vi "array.vi"() -> ()   [LabVIEW 2018]
panel:
  in  "数组 4":bool[](array[boolean])
  in  "数组 3":dbl[][](array[numeric])
  out "数组函数":i32[](array[numeric])
  in  "停止":bool
  out "数组 2":i32[](array[numeric])
  out "数组":i32[](array[numeric])
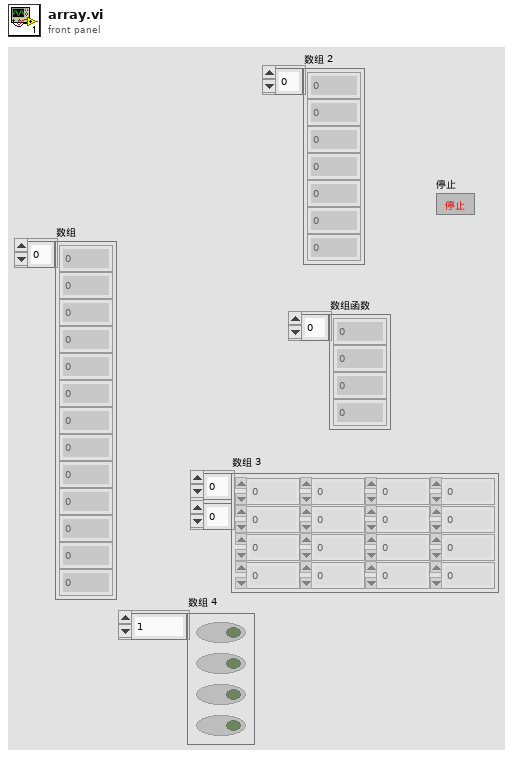
[diagram p1: front panel]
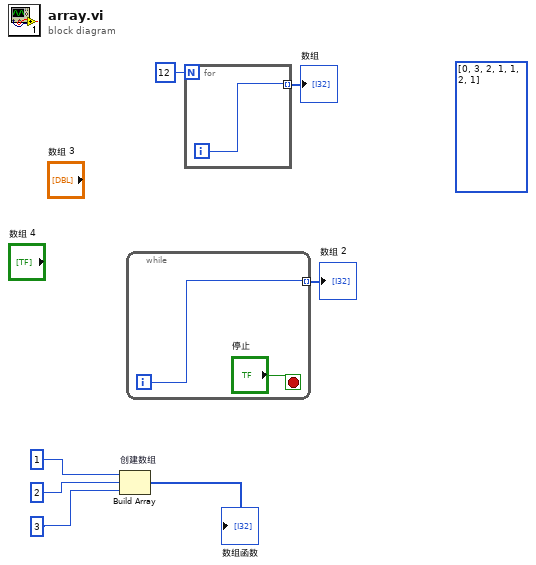
[diagram p0: block diagram]
diagram:
  (unwired) i32[] [0, 3, 2, 1, 1, 2, 1]
  n1 = Build Array "创建数组"(1, 2, 3) -> (→"数组函数":i32[])
  n2 = while {
    tunnel: [w9] -> w5 mode=indexing
    i -> [w9]
    stop <- "停止" stop-if-true
  }
  "数组 2" <- w5
  n3 = for {
    N: 12 -> [_]
    tunnel: [w10] -> w6 mode=indexing
    i -> [w10]
  }
  "数组" <- w6
